vi "IlmInfoSalvestaja.vi"() -> ()   [LabVIEW 2020]
uses:
  Downloads/visuaalprogrammeerimine/visuaalprogrammeerimine/Ilmajaamad.ctl
  Downloads/visuaalprogrammeerimine/visuaalprogrammeerimine/Ilmajaam.ctl
panel:
  in  "file path (use dialog)":path
  out "Array":T1
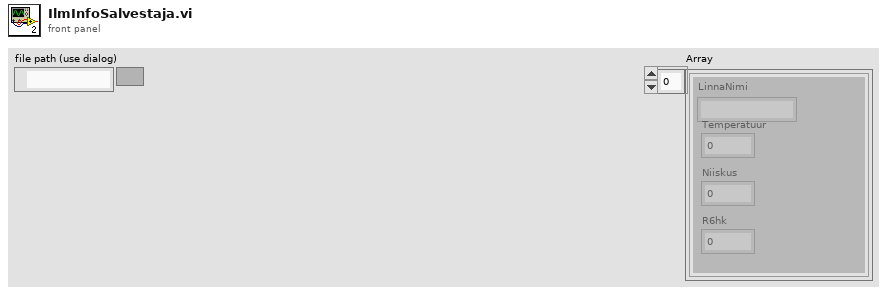
[diagram p1: front panel]
types:
  T1 = typedef "Ilmajaamad.ctl" = T2[]
  T2 = typedef "Ilmajaam.ctl" = cluster{"LinnaNimi":string, "Temperatuur":dbl, "Niiskus":dbl, "R6hk":dbl}
  T3 = enum16{"open", "replace", "create", "open or create", "replace or create", "replace or create with confirmation"}
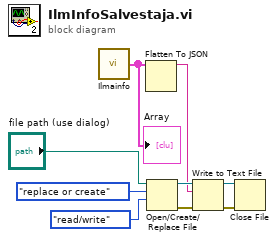
[diagram p0: block diagram]
diagram:
  n1 = call "Ilmainfo.vi"() -> ("Array"=w9:T1)
  "Array" <- w9
  n2 = Flatten To JSON(anything=w9) -> (JSON string=w3:string)  [unwired: 2 in, 1 out]
  n3 = Open/Create/Replace File(file path (use dialog)="file path (use dialog)", operation (0:open)=T3."replace or create", access (0:read/write)=enum16{"read/write", "read-only", "write-only"}."read/write") -> (refnum out=w7:refnum<file>, error out=w4:errorcluster)  [unwired: 3 in, 1 out]
  n4 = Write to Text File(file (use dialog)=w7, text=w3, error in=w4) -> (refnum out=w6:refnum<file>, error out=w5:errorcluster)  [unwired: 1 in, 1 out]
  n5 = Close File(refnum=w6, error in=w5) -> ()  [unwired: 2 out]
